vi "GeoData.vi"() -> ()   [LabVIEW 2017] (continued)
\t56033\tBig horn\tWY\tSheridan County\tH1\n82844\t56033\tWolf\tWY\tSheridan County\tH1\n82845\t56033\tWyarno\tWY\tSheridan County\tH1\n82836\t56033\tDayton\tWY\tSheridan County\tH1\n82842\t56033\tStory\tWY\tSheridan County\tH1\n82801\t56033\tSheridan\tWY\tSheridan County\tH1\n82837\t56033\tLeiter\tWY\tSheridan County\tH1\n82923\t56035\tBoulder\tWY\tSublette County\tH1\n82925\t56035\tCora\tWY\tSublette County\tH1\n83113\t56035\tBig piney\tWY\tSublette County\tH1\n82941\t56035\tPinedale\tWY\tSublette County\tH1\n83115\t56035\tDaniel\tWY\tSublette County\tH1\n82922\t56035\tBondurant\tWY\tSublette County\tH1\n82901\t56037\tRock springs\tWY\tSweetwater County\tH1\n82943\t56037\tReliance\tWY\tSweetwater County\tH1\n82929\t56037\tLittle america\tWY\tSweetwater County\tH1\n82336\t56037\tWamsutter\tWY\tSweetwater County\tH1\n82934\t56037\tGranger\tWY\tSweetwater County\tH1\n82902\t56037\tRock springs\tWY\tSweetwater County\tH1\n82935\t56037\tGreen river\tWY\tSweetwater County\tH1\n82322\t56037\tBairoil\tWY\tSweetwater County\tH1\n82945\t56037\tSuperior\tWY\tSweetwater County\tH1\n82932\t56037\tFarson\tWY\tSweetwater County\tH1\n82942\t56037\tPoint of rocks\tWY\tSweetwater County\tH1\n83002\t56039\tJackson\tWY\tTeton County\tH1\n82190\t56039\tYellowstone national park\tWY\tTeton County\tH1\n83014\t56039\tWilson\tWY\tTeton County\tH1\n83012\t56039\tMoose\tWY\tTeton County\tH1\n83013\t56039\tMoran\tWY\tTeton County\tH1\n83414\t56039\tAlta\tWY\tTeton County\tH1\n83001\t56039\tJackson\tWY\tTeton County\tH1\n83011\t56039\tKelly\tWY\tTeton County\tH1\n83025\t56039\tTeton village\tWY\tTeton County\tH1\n82931\t56041\tEvanston\tWY\tUinta County\tH1\n82939\t56041\tMountain view\tWY\tUinta County\tH1\n82930\t56041\tEvanston\tWY\tUinta County\tH1\n82933\t56041\tFort bridger\tWY\tUinta County\tH1\n82937\t56041\tLyman\tWY\tUinta County\tH1\n82944\t56041\tRobertson\tWY\tUinta County\tH1\n82936\t56041\tLonetree\tWY\tUinta County\tH1\n82442\t56043\tTen sleep\tWY\tWashakie County\tH1\n82401\t56043\tWorland\tWY\tWashakie County\tH1\n82701\t56045\tNewcastle\tWY\tWeston County\tH1\n82729\t56045\tSundance\tWY\tWeston County\tH1\n82723\t56045\tOsage\tWY\tWeston County\tH1\n82715\t56045\tFour corners\tWY\tWeston County\tH1\n82730\t56045\tUpton\tWY\tWeston County\tH1\n96910\t66010\tHagatna\tGU\tGuam\tH4\n96929\t66010\tYigo\tGU\tGuam\tH4\n96913\t66010\tBarrigada\tGU\tGuam\tH4\n96915\t66010\tSanta rita\tGU\tGuam\tH4\n601\t72001\tAdjuntas\tPR\tAdjuntas Municipio\tH1\n602\t72003\tAguada\tPR\tAguada Municipio\tH1\n603\t72005\tAguadilla\tPR\tAguadilla Municipio\tH1\n605\t72005\tAguadilla\tPR\tAguadilla Municipio\tH1\n690\t72005\tSan antonio\tPR\tAguadilla Municipio\tH1\n602\t72005\tAguada\tPR\tAguadilla Municipio\tH1\n604\t72005\tAguadilla\tPR\tAguadilla Municipio\tH1\n725\t72007\tCaguas\tPR\tAguas Buenas Municipio\tH1\n703\t72007\tAguas buenas\tPR\tAguas Buenas Municipio\tH1\n705\t72009\tAibonito\tPR\tAibonito Municipio\tH1\n786\t72009\tLa plata\tPR\tAibonito Municipio\tH1\n677\t72011\tRincon\tPR\tAnasco Municipio\tH1\n610\t72011\tAnasco\tPR\tAnasco Municipio\tH1\n652\t72013\tGarrochales\tPR\tArecibo Municipio\tH1\n614\t72013\tArecibo\tPR\tArecibo Municipio\tH1\n613\t72013\tArecibo\tPR\tArecibo Municipio\tH1\n650\t72013\tFlorida\tPR\tArecibo Municipio\tH1\n659\t72013\tHatillo\tPR\tArecibo Municipio\tH1\n612\t72013\tArecibo\tPR\tArecibo Municipio\tH1\n688\t72013\tSabana hoyos\tPR\tArecibo Municipio\tH1\n616\t72013\tBajadero\tPR\tArecibo Municipio\tH1\n714\t72015\tArroyo\tPR\tArroyo Municipio\tH1\n784\t72015\tGuayama\tPR\tArroyo Municipio\tH1\n617\t72017\tBarceloneta\tPR\tBarceloneta Municipio\tH1\n650\t72017\tFlorida\tPR\tBarceloneta Municipio\tH1\n794\t72019\tBarranquitas\tPR\tBarranquitas Municipio\tH1\n782\t72021\tComerio\tPR\tBayamon Municipio\tH1\n934\t72021\tFort buchanan\tPR\tBayamon Municipio\tH1\n917\t72021\tSan juan\tPR\tBayamon Municipio\tH1\n925\t72021\tSan juan\tPR\tBayamon Municipio\tH1\n920\t72021\tSan juan\tPR\tBayamon Municipio\tH1\n926\t72021\tSan juan\tPR\tBayamon Municipio\tH1\n962\t72021\tCatano\tPR\tBayamon Municipio\tH1\n921\t72021\tSan juan\tPR\tBayamon Municipio\tH1\n960\t72021\tBayamon\tPR\tBayamon Municipio\tH1\n969\t72021\tGuaynabo\tPR\tBayamon Municipio\tH1\n901\t72021\tSan juan\tPR\tBayamon Municipio\tH1\n949\t72021\tToa baja\tPR\tBayamon Municipio\tH1\n953\t72021\tToa alta\tPR\tBayamon Municipio\tH1\n961\t72021\tBayamon\tPR\tBayamon Municipio\tH1\n957\t72021\tBayamon\tPR\tBayamon Municipio\tH1\n976\t72021\tTrujillo alto\tPR\tBayamon Municipio\tH1\n924\t72021\tSan juan\tPR\tBayamon Municipio\tH1\n956\t72021\tBayamon\tPR\tBayamon Municipio\tH1\n959\t72021\tBayamon\tPR\tBayamon Municipio\tH1\n958\t72021\tBayamon\tPR\tBayamon Municipio\tH1\n622\t72023\tBoqueron\tPR\tCabo Rojo Municipio\tH1\n683\t72023\tSan german\tPR\tCabo Rojo Municipio\tH1\n623\t72023\tCabo rojo\tPR\tCabo Rojo Municipio\tH1\n667\t72023\tLajas\tPR\tCabo Rojo Municipio\tH1\n680\t72023\tMayaguez\tPR\tCabo Rojo Municipio\tH1\n725\t72025\tCaguas\tPR\tCaguas Municipio\tH1\n736\t72025\tCayey\tPR\tCaguas Municipio\tH1\n726\t72025\tCaguas\tPR\tCaguas Municipio\tH1\n754\t72025\tSan lorenzo\tPR\tCaguas Municipio\tH1\n926\t72025\tSan juan\tPR\tCaguas Municipio\tH1\n727\t72025\tCaguas\tPR\tCaguas Municipio\tH1\n778\t72025\tGurabo\tPR\tCaguas Municipio\tH1\n703\t72025\tAguas buenas\tPR\tCaguas Municipio\tH1\n723\t72025\tPatillas\tPR\tCaguas Municipio\tH1\n739\t72025\tCidra\tPR\tCaguas Municipio\tH1\n956\t72025\tBayamon\tPR\tCaguas Municipio\tH1\n627\t72027\tCamuy\tPR\tCamuy Municipio\tH1\n777\t72029\tJuncos\tPR\tCanovanas Municipio\tH1\n745\t72029\tRio grande\tPR\tCanovanas Municipio\tH1\n729\t72029\tCanovanas\tPR\tCanovanas Municipio\tH1\n979\t72029\tCarolina\tPR\tCanovanas Municipio\tH1\n778\t72029\tGurabo\tPR\tCanovanas Municipio\tH1\n987\t72029\tCarolina\tPR\tCanovanas Municipio\tH1\n985\t72031\tCarolina\tPR\tCarolina Municipio\tH1\n984\t72031\tCarolina\tPR\tCarolina Municipio\tH1\n986\t72031\tCarolina\tPR\tCarolina Municipio\tH1\n926\t72031\tSan juan\tPR\tCarolina Municipio\tH1\n983\t72031\tCarolina\tPR\tCarolina Municipio\tH1\n921\t72031\tSan juan\tPR\tCarolina Municipio\tH1\n937\t72031\tSan juan\tPR\tCarolina Municipio\tH1\n729\t72031\tCanovanas\tPR\tCarolina Municipio\tH1\n979\t72031\tCarolina\tPR\tCarolina Municipio\tH1\n778\t72031\tGurabo\tPR\tCarolina Municipio\tH1\n976\t72031\tTrujillo alto\tPR\tCarolina Municipio\tH1\n988\t72031\tCarolina\tPR\tCarolina Municipio\tH1\n981\t72031\tCarolina\tPR\tCarolina Municipio\tH1\n924\t72031\tSan juan\tPR\tCarolina Municipio\tH1\n959\t72031\tBayamon\tPR\tCarolina Municipio\tH1\n982\t72031\tCarolina\tPR\tCarolina Municipio\tH1\n987\t72031\tCarolina\tPR\tCarolina Municipio\tH1\n977\t72033\tTrujillo alto\tPR\tCatano Municipio\tH1\n917\t72033\tSan juan\tPR\tCatano Municipio\tH1\n920\t72033\tSan juan\tPR\tCatano Municipio\tH1\n926\t72033\tSan juan\tPR\tCatano Municipio\tH1\n962\t72033\tCatano\tPR\tCatano Municipio\tH1\n949\t72033\tToa baja\tPR\tCatano Municipio\tH1\n778\t72033\tGurabo\tPR\tCatano Municipio\tH1\n961\t72033\tBayamon\tPR\tCatano Municipio\tH1\n909\t72033\tSan juan\tPR\tCatano Municipio\tH1\n957\t72033\tBayamon\tPR\tCatano Municipio\tH1\n976\t72033\tTrujillo alto\tPR\tCatano Municipio\tH1\n963\t72033\tCatano\tPR\tCatano Municipio\tH1\n956\t72033\tBayamon\tPR\tCatano Municipio\tH1\n959\t72033\tBayamon\tPR\tCatano Municipio\tH1\n736\t72035\tCayey\tPR\tCayey Municipio\tH1\n754\t72035\tSan lorenzo\tPR\tCayey Municipio\tH1\n737\t72035\tCayey\tPR\tCayey Municipio\tH1\n705\t72035\tAibonito\tPR\tCayey Municipio\tH1\n739\t72035\tCidra\tPR\tCayey Municipio\tH1\n735\t72037\tCeiba\tPR\tCeiba Municipio\tH1\n738\t72037\tFajardo\tPR\tCeiba Municipio\tH1\n742\t72037\tRoosevelt roads\tPR\tCeiba Municipio\tH1\n638\t72039\tCiales\tPR\tCiales Municipio\tH1\n725\t72041\tCaguas\tPR\tCidra Municipio\tH1\n739\t72041\tCidra\tPR\tCidra Municipio\tH1\n769\t72043\tCoamo\tPR\tCoamo Municipio\tH1\n705\t72043\tAibonito\tPR\tCoamo Municipio\tH1\n782\t72045\tComerio\tPR\tComerio Municipio\tH1\n783\t72047\tCorozal\tPR\tCorozal Municipio\tH1\n794\t72047\tBarranquitas\tPR\tCorozal Municipio\tH1\n775\t72049\tCulebra\tPR\tCulebra Municipio\tH1\n646\t72051\tDorado\tPR\tDorado Municipio\tH1\n949\t72051\tToa baja\tPR\tDorado Municipio\tH1\n692\t72051\tVega alta\tPR\tDorado Municipio\tH1\n735\t72053\tCeiba\tPR\tFajardo Municipio\tH1\n738\t72053\tFajardo\tPR\tFajardo Municipio\tH1\n740\t72053\tPuerto real\tPR\tFajardo Municipio\tH1\n617\t72054\tBarceloneta\tPR\tFlorida Municipio\tH1\n650\t72054\tFlorida\tPR\tFlorida Municipio\tH1\n612\t72054\tArecibo\tPR\tFlorida Municipio\tH1\n653\t72055\tGuanica\tPR\tGuanica Municipio\tH1\n647\t72055\tEnsenada\tPR\tGuanica Municipio\tH1\n714\t72057\tArroyo\tPR\tGuayama Municipio\tH1\n785\t72057\tGuayama\tPR\tGuayama Municipio\tH1\n784\t72057\tGuayama\tPR\tGuayama Municipio\tH1\n723\t72057\tPatillas\tPR\tGuayama Municipio\tH1\n624\t72059\tPenuelas\tPR\tGuayanilla Municipio\tH1\n656\t72059\tGuayanilla\tPR\tGuayanilla Municipio\tH1\n934\t72061\tFort buchanan\tPR\tGuaynabo Municipio\tH1\n965\t72061\tGuaynabo\tPR\tGuaynabo Municipio\tH1\n917\t72061\tSan juan\tPR\tGuaynabo Municipio\tH1\n971\t72061\tGuaynabo\tPR\tGuaynabo Municipio\tH1\n920\t72061\tSan juan\tPR\tGuaynabo Municipio\tH1\n926\t72061\tSan juan\tPR\tGuaynabo Municipio\tH1\n962\t72061\tCatano\tPR\tGuaynabo Municipio\tH1\n922\t72061\tSan juan\tPR\tGuaynabo Municipio\tH1\n921\t72061\tSan juan\tPR\tGuaynabo Municipio\tH1\n969\t72061\tGuaynabo\tPR\tGuaynabo Municipio\tH1\n970\t72061\tGuaynabo\tPR\tGuaynabo Municipio\tH1\n968\t72061\tGuaynabo\tPR\tGuaynabo Municipio\tH1\n966\t72061\tGuaynabo\tPR\tGuaynabo Municipio\tH1\n959\t72061\tBayamon\tPR\tGuaynabo Municipio\tH1\n725\t72063\tCaguas\tPR\tGurabo Municipio\tH1\n777\t72063\tJuncos\tPR\tGurabo Municipio\tH1\n754\t72063\tSan lorenzo\tPR\tGurabo Municipio\tH1\n729\t72063\tCanovanas\tPR\tGurabo Municipio\tH1\n778\t72063\tGurabo\tPR\tGurabo Municipio\tH1\n659\t72065\tHatillo\tPR\tHatillo Municipio\tH1\n612\t72065\tArecibo\tPR\tHatillo Municipio\tH1\n660\t72067\tHormigueros\tPR\tHormigueros Municipio\tH1\n680\t72067\tMayaguez\tPR\tHormigueros Municipio\tH1\n791\t72069\tHumacao\tPR\tHumacao Municipio\tH1\n741\t72069\tPunta santiago\tPR\tHumacao Municipio\tH1\n792\t72069\tHumacao\tPR\tHumacao Municipio\tH1\n603\t72071\tAguadilla\tPR\tIsabela Municipio\tH1\n690\t72071\tSan antonio\tPR\tIsabela Municipio\tH1\n662\t72071\tIsabela\tPR\tIsabela Municipio\tH1\n664\t72073\tJayuya\tPR\tJayuya Municipio\tH1\n766\t72075\tVillalba\tPR\tJuana Diaz Municipio\tH1\n795\t72075\tJuana diaz\tPR\tJuana Diaz Municipio\tH1\n720\t72075\tOrocovis\tPR\tJuana Diaz Municipio\tH1\n777\t72077\tJuncos\tPR\tJuncos Municipio\tH1\n778\t72077\tGurabo\tPR\tJuncos Municipio\tH1\n683\t72079\tSan german\tPR\tLajas Municipio\tH1\n667\t72079\tLajas\tPR\tLajas Municipio\tH1\n669\t72081\tLares\tPR\tLares Municipio\tH1\n631\t72081\tCastaner\tPR\tLares Municipio\tH1\n670\t72083\tLas marias\tPR\tLas Marias Municipio\tH1\n771\t72085\tLas piedras\tPR\tLas Piedras Municipio\tH1\n772\t72087\tLoiza\tPR\tLoiza Municipio\tH1\n745\t72087\tRio grande\tPR\tLoiza Municipio\tH1\n729\t72087\tCanovanas\tPR\tLoiza Municipio\tH1\n773\t72089\tLuquillo\tPR\tLuquillo Municipio\tH1\n674\t72091\tManati\tPR\tManati Municipio\tH1\n687\t72091\tMorovis\tPR\tManati Municipio\tH1\n650\t72091\tFlorida\tPR\tManati Municipio\tH1\n638\t72091\tCiales\tPR\tManati Municipio\tH1\n693\t72091\tVega baja\tPR\tManati Municipio\tH1\n606\t72093\tMaricao\tPR\tMaricao Municipio\tH1\n707\t72095\tMaunabo\tPR\tMaunabo Municipio\tH1\n682\t72097\tMayaguez\tPR\tMayaguez Municipio\tH1\n681\t72097\tMayaguez\tPR\tMayaguez Municipio\tH1\n683\t72097\tSan german\tPR\tMayaguez Municipio\tH1\n660\t72097\tHormigueros\tPR\tMayaguez Municipio\tH1\n623\t72097\tCabo rojo\tPR\tMayaguez Municipio\tH1\n680\t72097\tMayaguez\tPR\tMayaguez Municipio\tH1\n676\t72099\tMoca\tPR\tMoca Municipio\tH1\n603\t72099\tAguadilla\tPR\tMoca Municipio\tH1\n685\t72099\tSan sebastian\tPR\tMoca Municipio\tH1\n674\t72101\tManati\tPR\tMorovis Municipio\tH1\n687\t72101\tMorovis\tPR\tMorovis Municipio\tH1\n692\t72101\tVega alta\tPR\tMorovis Municipio\tH1\n720\t72101\tOrocovis\tPR\tMorovis Municipio\tH1\n718\t72103\tNaguabo\tPR\tNaguabo Municipio\tH1\n744\t72103\tRio blanco\tPR\tNaguabo Municipio\tH1\n771\t72103\tLas piedras\tPR\tNaguabo Municipio\tH1\n719\t72105\tNaranjito\tPR\tNaranjito Municipio\tH1\n720\t72107\tOrocovis\tPR\tOrocovis Municipio\tH1\n638\t72107\tCiales\tPR\tOrocovis Municipio\tH1\n723\t72109\tPatillas\tPR\tPatillas Municipio\tH1\n624\t72111\tPenuelas\tPR\tPenuelas Municipio\tH1\n731\t72113\tPonce\tPR\tPonce Municipio\tH1\n780\t72113\tCoto laurel\tPR\tPonce Municipio\tH1\n641\t72113\tUtuado\tPR\tPonce Municipio\tH1\n730\t72113\tPonce\tPR\tPonce Municipio\tH1\n732\t72113\tPonce\tPR\tPonce Municipio\tH1\n733\t72113\tPonce\tPR\tPonce Municipio\tH1\n715\t72113\tMercedita\tPR\tPonce Municipio\tH1\n728\t72113\tPonce\tPR\tPonce Municipio\tH1\n795\t72113\tJuana diaz\tPR\tPonce Municipio\tH1\n601\t72113\tAdjuntas\tPR\tPonce Municipio\tH1\n624\t72113\tPenuelas\tPR\tPonce Municipio\tH1\n717\t72113\tPonce\tPR\tPonce Municipio\tH1\n716\t72113\tPonce\tPR\tPonce Municipio\tH1\n678\t72115\tQuebradillas\tPR\tQuebradillas Municipio\tH1\n662\t72115\tIsabela\tPR\tQuebradillas Municipio\tH1\n677\t72117\tRincon\tPR\tRincon Municipio\tH1\n721\t72119\tPalmer\tPR\tRio Grande Municipio\tH1\n735\t72119\tCeiba\tPR\tRio Grande Municipio\tH1\n745\t72119\tRio grande\tPR\tRio Grande Municipio\tH1\n698\t72121\tYauco\tPR\tSabana Grande Municipio\tH1\n637\t72121\tSabana grande\tPR\tSabana Grande Municipio\tH1\n647\t72121\tEnsenada\tPR\tSabana Grande Municipio\tH1\n757\t72123\tSanta isabel\tPR\tSalinas Municipio\tH1\n751\t72123\tSalinas\tPR\tSalinas Municipio\tH1\n704\t72123\tAguirre\tPR\tSalinas Municipio\tH1\n683\t72125\tSan german\tPR\tSan German Municipio\tH1\n725\t72127\tCaguas\tPR\tSan Juan Municipio\tH1\n782\t72127\tComerio\tPR\tSan Juan Municipio\tH1\n902\t72127\tSan juan\tPR\tSan Juan Municipio\tH1\n918\t72127\tSan juan\tPR\tSan Juan Municipio\tH1\n917\t72127\tSan juan\tPR\tSan Juan Municipio\tH1\n925\t72127\tSan juan\tPR\tSan Juan Municipio\tH1\n971\t72127\tGuaynabo\tPR\tSan Juan Municipio\tH1\n940\t72127\tSan juan\tPR\tSan Juan Municipio\tH1\n908\t72127\tSan juan\tPR\tSan Juan Municipio\tH1\n923\t72127\tSan juan\tPR\tSan Juan Municipio\tH1\n920\t72127\tSan juan\tPR\tSan Juan Municipio\tH1\n926\t72127\tSan juan\tPR\tSan Juan Municipio\tH1\n936\t72127\tSan juan\tPR\tSan Juan Municipio\tH1\n931\t72127\tSan juan\tPR\tSan Juan Municipio\tH1\n962\t72127\tCatano\tPR\tSan Juan Municipio\tH1\n928\t72127\tSan juan\tPR\tSan Juan Municipio\tH1\n912\t72127\tSan juan\tPR\tSan Juan Municipio\tH1\n910\t72127\tSan juan\tPR\tSan Juan Municipio\tH1\n921\t72127\tSan juan\tPR\tSan Juan Municipio\tH1\n969\t72127\tGuaynabo\tPR\tSan Juan Municipio\tH1\n901\t72127\tSan juan\tPR\tSan Juan Municipio\tH1\n975\t72127\tSan juan\tPR\tSan Juan Municipio\tH1\n778\t72127\tGurabo\tPR\tSan Juan Municipio\tH1\n907\t72127\tSan juan\tPR\tSan Juan Municipio\tH1\n913\t72127\tSan juan\tPR\tSan Juan Municipio\tH1\n919\t72127\tSan juan\tPR\tSan Juan Municipio\tH1\n927\t72127\tSan juan\tPR\tSan Juan Municipio\tH1\n961\t72127\tBayamon\tPR\tSan Juan Municipio\tH1\n968\t72127\tGuaynabo\tPR\tSan Juan Municipio\tH1\n719\t72127\tNaranjito\tPR\tSan Juan Municipio\tH1\n911\t72127\tSan juan\tPR\tSan Juan Municipio\tH1\n909\t72127\tSan juan\tPR\tSan Juan Municipio\tH1\n957\t72127\tBayamon\tPR\tSan Juan Municipio\tH1\n976\t72127\tTrujillo alto\tPR\tSan Juan Municipio\tH1\n929\t72127\tSan juan\tPR\tSan Juan Municipio\tH1\n935\t72127\tSan juan\tPR\tSan Juan Municipio\tH1\n915\t72127\tSan juan\tPR\tSan Juan Municipio\tH1\n924\t72127\tSan juan\tPR\tSan Juan Municipio\tH1\n956\t72127\tBayamon\tPR\tSan Juan Municipio\tH1\n959\t72127\tBayamon\tPR\tSan Juan Municipio\tH1\n987\t72127\tCarolina\tPR\tSan Juan Municipio\tH1\n914\t72127\tSan juan\tPR\tSan Juan Municipio\tH1\n916\t72127\tSan juan\tPR\tSan Juan Municipio\tH1\n725\t72129\tCaguas\tPR\tSan Lorenzo Municipio\tH1\n754\t72129\tSan lorenzo\tPR\tSan Lorenzo Municipio\tH1\n771\t72129\tLas piedras\tPR\tSan Lorenzo Municipio\tH1\n778\t72129\tGurabo\tPR\tSan Lorenzo Municipio\tH1\n685\t72131\tSan sebastian\tPR\tSan Sebastian Municipio\tH1\n757\t72133\tSanta isabel\tPR\tSanta Isabel Municipio\tH1\n751\t72133\tSalinas\tPR\tSanta Isabel Municipio\tH1\n646\t72135\tDorado\tPR\tToa Alta Municipio\tH1\n783\t72135\tCorozal\tPR\tToa Alta Municipio\tH1\n954\t72135\tToa alta\tPR\tToa Alta Municipio\tH1\n949\t72135\tToa baja\tPR\tToa Alta Municipio\tH1\n692\t72135\tVega alta\tPR\tToa Alta Municipio\tH1\n953\t72135\tToa alta\tPR\tToa Alta Municipio\tH1\n957\t72135\tBayamon\tPR\tToa Alta Municipio\tH1\n951\t72137\tToa baja\tPR\tToa Baja Municipio\tH1\n646\t72137\tDorado\tPR\tToa Baja Municipio\tH1\n952\t72137\tSabana seca\tPR\tToa Baja Municipio\tH1\n949\t72137\tToa baja\tPR\tToa Baja Municipio\tH1\n950\t72137\tToa baja\tPR\tToa Baja Municipio\tH1\n953\t72137\tToa alta\tPR\tToa Baja Municipio\tH1\n961\t72137\tBayamon\tPR\tToa Baja Municipio\tH1\n917\t72139\tSan juan\tPR\tTrujillo Alto Municipio\tH1\n926\t72139\tSan juan\tPR\tTrujillo Alto Municipio\tH1\n962\t72139\tCatano\tPR\tTrujillo Alto Municipio\tH1\n969\t72139\tGuaynabo\tPR\tTrujillo Alto Municipio\tH1\n949\t72139\tToa baja\tPR\tTrujillo Alto Municipio\tH1\n778\t72139\tGurabo\tPR\tTrujillo Alto Municipio\tH1\n961\t72139\tBayamon\tPR\tTrujillo Alto Municipio\tH1\n957\t72139\tBayamon\tPR\tTrujillo Alto Municipio\tH1\n976\t72139\tTrujillo alto\tPR\tTrujillo Alto Municipio\tH1\n924\t72139\tSan juan\tPR\tTrujillo Alto Municipio\tH1\n956\t72139\tBayamon\tPR\tTrujillo Alto Municipio\tH1\n959\t72139\tBayamon\tPR\tTrujillo Alto Municipio\tH1\n987\t72139\tCarolina\tPR\tTrujillo Alto Municipio\tH1\n641\t72141\tUtuado\tPR\tUtuado Municipio\tH1\n612\t72141\tArecibo\tPR\tUtuado Municipio\tH1\n611\t72141\tAngeles\tPR\tUtuado Municipio\tH1\n646\t72143\tDorado\tPR\tVega Alta Municipio\tH1\n687\t72143\tMorovis\tPR\tVega Alta Municipio\tH1\n692\t72143\tVega alta\tPR\tVega Alta Municipio\tH1\n693\t72143\tVega baja\tPR\tVega Alta Municipio\tH1\n674\t72145\tManati\tPR\tVega Baja Municipio\tH1\n687\t72145\tMorovis\tPR\tVega Baja Municipio\tH1\n692\t72145\tVega alta\tPR\tVega Baja Municipio\tH1\n693\t72145\tVega baja\tPR\tVega Baja Municipio\tH1\n694\t72145\tVega baja\tPR\tVega Baja Municipio\tH1\n765\t72147\tVieques\tPR\tVieques Municipio\tH1\n766\t72149\tVillalba\tPR\tVillalba Municipio\tH1\n720\t72149\tOrocovis\tPR\tVillalba Municipio\tH1\n767\t72151\tYabucoa\tPR\tYabucoa Municipio\tH1\n606\t72153\tMaricao\tPR\tYauco Municipio\tH1\n698\t72153\tYauco\tPR\tYauco Municipio\tH1\n653\t72153\tGuanica\tPR\tYauco Municipio\tH1\n820\t78010\tChristiansted\tVI\tSt. Croix Island\tH4\n840\t78010\tFrederiksted\tVI\tSt. Croix Island\tH4\n850\t78010\tKingshill\tVI\tSt. Croix Island\tH4\n830\t78020\tSt john\tVI\tSt. John Island\tH4\n802\t78030\tSt thomas\tVI\tSt. Thomas Island\tH4\n", array type (2D Dbl)=string[][] []) -> (array=w31:string[][])  [unwired: 1 in]
  n2 = Spreadsheet String To Array(format string="%s", spreadsheet string="1\tAL\tAlabama\t1779775\n2\tAK\tAlaska\t1785533\n4\tAZ\tArizona\t1779777\n5\tAR\tArkansas\t68085\n6\tCA\tCalifornia\t1779778\n8\tCO\tColorado\t1779779\n9\tCT\tConnecticut\t1779780\n10\tDE\tDelaware\t1779781\n11\tDC\tDistrict of Columbia\t1702382\n12\tFL\tFlorida\t294478\n13\tGA\tGeorgia\t1705317\n15\tHI\tHawaii\t1779782\n16\tID\tIdaho\t1779783\n17\tIL\tIllinois\t1779784\n18\tIN\tIndiana\t448508\n19\tIA\tIowa\t1779785\n20\tKS\tKansas\t481813\n21\tKY\tKentucky\t1779786\n22\tLA\tLouisiana\t1629543\n23\tME\tMaine\t1779787\n24\tMD\tMaryland\t1714934\n25\tMA\tMassachusetts\t606926\n26\tMI\tMichigan\t1779789\n27\tMN\tMinnesota\t662849\n28\tMS\tMississippi\t1779790\n29\tMO\tMissouri\t1779791\n30\tMT\tMontana\t767982\n31\tNE\tNebraska\t1779792\n32\tNV\tNevada\t1779793\n33\tNH\tNew Hampshire\t1779794\n34\tNJ\tNew Jersey\t1779795\n35\tNM\tNew Mexico\t897535\n36\tNY\tNew York\t1779796\n37\tNC\tNorth Carolina\t1027616\n38\tND\tNorth Dakota\t1779797\n39\tOH\tOhio\t1085497\n40\tOK\tOklahoma\t1102857\n41\tOR\tOregon\t1155107\n42\tPA\tPennsylvania\t1779798\n44\tRI\tRhode Island\t1219835\n45\tSC\tSouth Carolina\t1779799\n46\tSD\tSouth Dakota\t1785534\n47\tTN\tTennessee\t1325873\n48\tTX\tTexas\t1779801\n49\tUT\tUtah\t1455989\n50\tVT\tVermont\t1779802\n51\tVA\tVirginia\t1779803\n53\tWA\tWashington\t1779804\n54\tWV\tWest Virginia\t1779805\n55\tWI\tWisconsin\t1779806\n56\tWY\tWyoming\t1779807\n60\tAS\tAmerican Samoa\t1802701\n66\tGU\tGuam\t1802705\n69\tMP\tNorthern Mariana Islands\t1779809\n72\tPR\tPuerto Rico\t1779808\n74\tUM\tU.S. Minor Outlying Islands\t1878752\n78\tVI\tU.S. Virgin Islands\t1802710\n", array type (2D Dbl)=string[][] []) -> (array=w13:string[][])  [unwired: 1 in]
  n3 = Index Array(array=w31, index (col) #1=0 ("disabled index (col)"), index (col) #2=1 ("index (col)"), index (col) #3=2 ("index (col)"), index (col) #4=3 ("index (col)"), index (col) #5=4 ("index (col)")) -> (element #1=w30:string[], element #2=w28:string[], element #3=→"City":string[], element #4=w7:string[], element #5=→"County":string[])  [unwired: 5 in]
  "State" <- w7
  n4 = Index Array(array=w13, index (col) #1=0 ("disabled index (col)"), index (col) #2=1 ("index (col)"), index (col) #3=2 ("index (col)"), index (col) #4=3 ("index (col)")) -> (element #1=w10:string[], element #2=w8:string[], element #3=w6:string[], element #4=w9:string[])  [unwired: 4 in]
  n5 = Decimal String To Number(string=w30) -> (number=→"Zip":i32[])  [unwired: 2 in, 1 out]
  n6 = Decimal String To Number(string=w28) -> (number=→"Fips":i32[])  [unwired: 2 in, 1 out]
  n7 = Decimal String To Number(string=w10) -> (number=w2:i32[])  [unwired: 2 in, 1 out]
  n8 = Decimal String To Number(string=w9) -> (number=w5:i32[])  [unwired: 2 in, 1 out]
  n9 = for {
    tunnel: w8 -> [w42]
    tunnel: w7 -> [w41] mode=indexing
    tunnel: w6 -> [w40]
    tunnel: [w39] -> w4 mode=indexing
    tunnel: w5 -> [w37]
    tunnel: [w38] -> w3 mode=indexing
    tunnel: w2 -> [w36]
    tunnel: [w34] -> w1 mode=indexing
    n10 = Search 1D Array(1D array=w42, element=w41) -> (index of element=w35:i32)  [unwired: 1 in]
    n11 = Index Array(array=w40, index=w35) -> (element=w39:string)
    n12 = Index Array(array=w37, index=w35) -> (element=w38:i32)
    n13 = Index Array(array=w36, index=w35) -> (element=w34:i32)
  }
  "StateName" <- w4
  "EINS" <- w3
  "StateFIPS" <- w1
